vi "Append User Formatted HTML to Report.vi"(0 "report in":refnum<class "NI_report.lvclass">, 5 "HTML text":string, 11 "error in (no error)":errorcluster) -> (4 "report out":refnum<class "NI_report.lvclass">, 15 "error out":errorcluster)   [LabVIEW 2017, in "NI_report.lvclass"]
doc: "Inserts text that is not preformatted by LabVIEW in the HTML report. You cannot use this VI with standard reports."
uses:
  <vilib>/Utility/NIReport.llb/NI_report.lvclass
  <vilib>/Utility/NIReport.llb/NI_ReportGenerationCore.lvlib
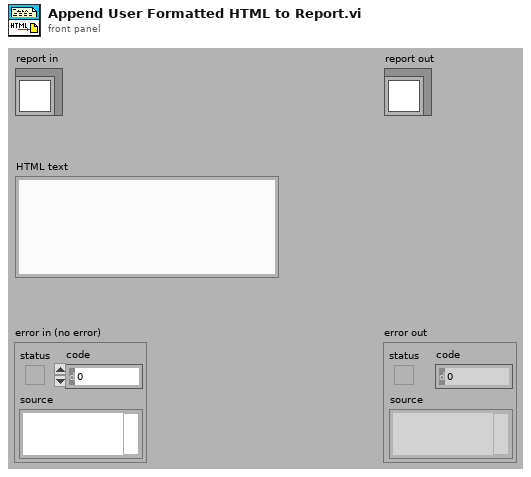
[diagram p1: front panel]
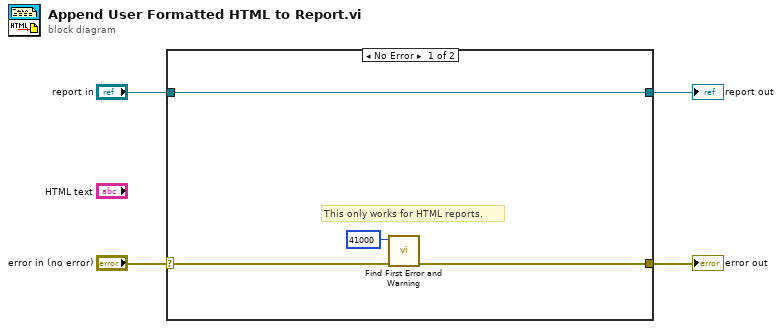
[diagram p0: block diagram]
diagram:
  n1 = case shown="No Error" "error in (no error)" {
    selector: "error in (no error)" -> [w6 w10]
    tunnel: [w5 w10] -> w3
    tunnel: [w8 w9] -> w1
    tunnel: "report in" -> [w8 w9]
    frame No Error {
      # "This only works for HTML reports."
      n2 = call <vilib>:"Find First Error and Warning.vi"("error in (no error)"=w6, "error code"=41000) -> ("error out"=w5:errorcluster)  [unwired: 1 in, 4 out]
    }
    frame Error {
    }
  }
  "error out" <- w3
  "report out" <- w1
